vi "PopUp_About.vi"(8 "error in (no error)":errorcluster) -> (0 "error out":errorcluster)   [LabVIEW 2013, in "SET Project Editor.lvlib"]
uses:
  SET Project Editor.lvlib
  DialogEnum.ctl
panel:
  in  "OK":bool
  # "SET Toolkit"
  # "Version 0.4.0"
  # "Copyright © 2014, Ryan Porter\nAll rights reserved."
  # "The SET Toolkit has been developed to provide more convenient edit-time language\nswitching for LabVIEW projects."
  # "Distributed under the BSD 2-Clause (http://opensource.org/licenses/BSD-2-Clause)"
  # "Developed using National Instruments LabVIEW\"!  2013."
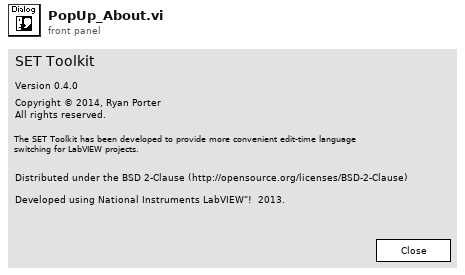
[diagram p1: front panel]
types:
  T1 = typedef "SET Project Editor.lvlib/DialogEnum.ctl" = enum16{"Idle", "Init", "Shutdown"}
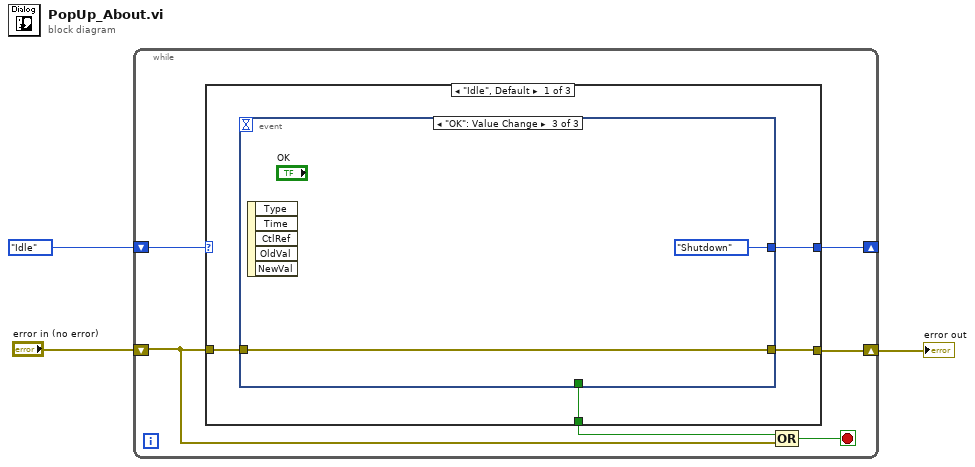
[diagram p0: block diagram]
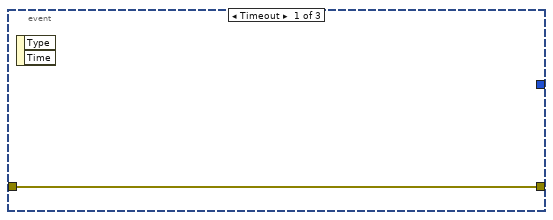
[diagram p2: hidden frame]
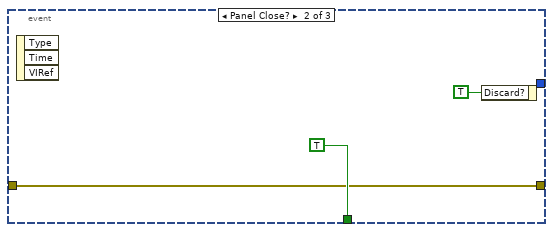
[diagram p3: hidden frame]
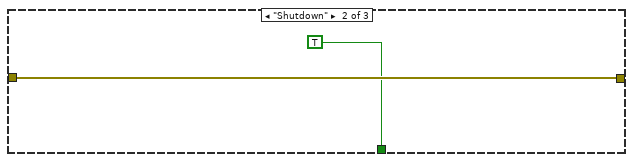
[diagram p4: hidden frame]
diagram:
  n1 = while {
    shift-right: [w8] -> w1
    shift-left: "error in (no error)" -> [w5]
    shift-right: [w7] -> _
    shift-left: DialogEnum."Idle" -> [w9]
    stop <- w4 stop-if-true
    n2 = case shown="\"Idle\", Default" w9 {
      tunnel: [w13 w21 w22] -> w8
      tunnel: w5 -> [w12 w21 w22]
      tunnel: [w11 TRUE _] -> w6
      tunnel: [w10 _ _] -> w7
      frame "Idle", Default {
        n3 = event shown="[2] \"OK\": Value Change" {
          selector: _ -> [_ _ _]
          dyn-events: _ -> [_ _ _]
          timeout: _ -> [_ _ _]
          tunnel: [w14 w15 w18] -> w13
          tunnel: w12 -> [w14 w15 w18]
          tunnel: [_ TRUE _] -> w11
          tunnel: [_ _ DialogEnum."Shutdown"] -> w10
          event Timeout {
            n4 = event-data() -> ()  [unwired: 1 in, 2 out]
          }
          event Panel Close? {
            n5 = event-data() -> ()  [unwired: 1 in, 3 out]
            n6 = event-data("Discard?"=TRUE) -> ()  [unwired: 1 in, 1 out]
          }
          event "OK": Value Change {
            n7 = event-data() -> ()  [unwired: 1 in, 5 out]
          }
        }
      }
      frame "Shutdown" {
      }
      frame "Init" {
      }
    }
    n8 = Compound Arithmetic op=OR(w6, w5) -> (w4:bool)
  }
  "error out" <- w1
